vi "coordinate.vi"() -> ()   [LabVIEW 2018]
uses:
  <vilib>/MediaMongrels Ltd/WebSockets/WebSockets/WebSocket Client/WebSocket Client.lvclass
  D:/software_setup/National Instruments/LabVIEW 2018/vi.lib/MediaMongrels Ltd/WebSockets/WebSockets/WebSocket/WebSocket.lvclass
panel:
  out "xyzr 2":dbl[](array[numeric])
  out "xyzr":dbl[](array[numeric])
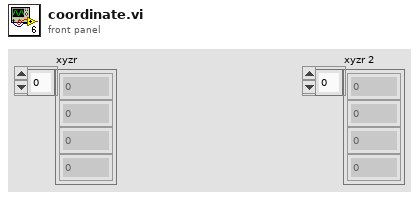
[diagram p1: front panel]
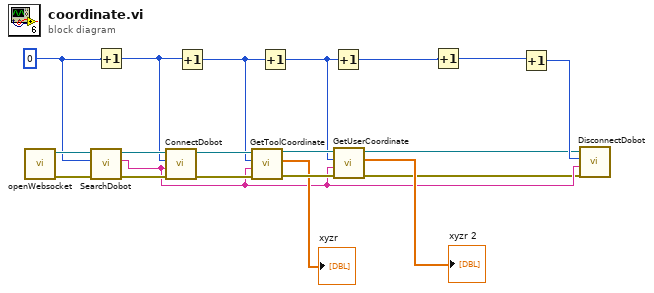
[diagram p0: block diagram]
diagram:
  w16 = 0 ("id")
  n1 = call <vilib>:"openWebsocket.vi"() -> ("error out"=w18:errorcluster, "WebSocket Client out"=w20:refnum<class "WebSocket Client.lvclass">)  [unwired: 10 in]
  n2 = call <vilib>:"SearchDobot.vi"("error in (no error)"=w18, "id"=w16, "WebSocket in"=w20) -> ("error out"=w17:errorcluster, "portName"=w3:string, "WebSocket out"=w19:refnum<class "WebSocket Client.lvclass">)  [unwired: 6 in]
  n3 = Increment(x=w16) -> (x+1=w15:i32)
  n4 = call <vilib>:"ConnectDobot.vi"("error in (no error)"=w17, "portName"=w3, "id"=w15, "WebSocket in"=w19) -> ("error out"=w10:errorcluster, "WebSocket out"=w11:refnum<class "WebSocket Client.lvclass">)  [unwired: 5 in, 1 out]
  n5 = Increment(x=w15) -> (x+1=w5:i32)
  n6 = call <vilib>:"GetToolCoordinate.vi"("error in (no error)"=w10, "portName"=w3, "id"=w5, "WebSocket in"=w11) -> ("error out"=w8:errorcluster, "xyzr"=→"xyzr":dbl[], "WebSocket out"=w9:refnum<class "WebSocket Client.lvclass">)  [unwired: 5 in]
  n7 = Increment(x=w5) -> (x+1=w4:i32)
  n8 = Increment(x=w4) -> (x+1=w13:i32)
  n9 = call <vilib>:"GetUserCoordinate.vi"("error in (no error)"=w8, "portName"=w3, "id"=w4, "WebSocket in"=w9) -> ("error out"=w1:errorcluster, "xyzr"=→"xyzr 2":dbl[], "WebSocket out"=w2:refnum<class "WebSocket Client.lvclass">)  [unwired: 5 in]
  n10 = Increment(x=w13) -> (x+1=w12:i32)
  n11 = Increment(x=w12) -> (x+1=w14:i32)
  n12 = call <vilib>:"DisconnectDobot.vi"("error in (no error)"=w1, "portName"=w3, "id"=w14, "WebSocket in"=w2) -> ()  [unwired: 5 in, 3 out]
